vi "Read Line.vi"(8 "error in (no error)":errorcluster, 11 "Table Manager in":refnum<class "Table Manager.lvclass">) -> (0 "error out":errorcluster, 2 "Table Manager.lvlib:Line.lvclass":refnum<class "Line.lvclass">, 3 "Table Manager out":refnum<class "Table Manager.lvclass">)   [LabVIEW 2013, in "Table Manager.lvlib" / "Table Manager.lvclass"]
uses:
  Table Manager.lvclass
  Line/Line.lvclass
  Table Manager.lvclass/Table Manager.ctl
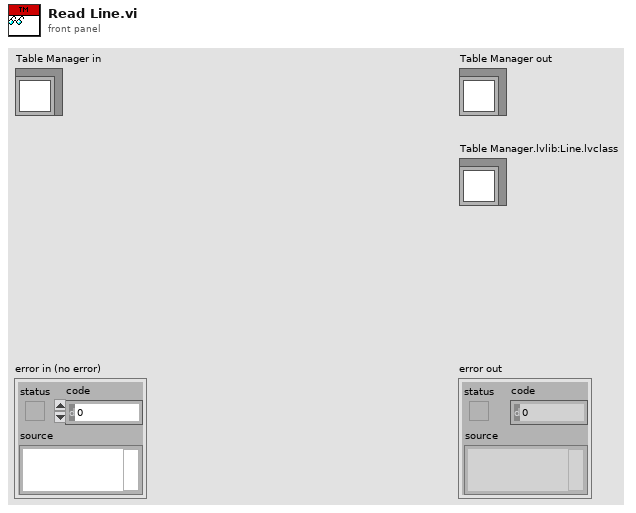
[diagram p1: front panel]
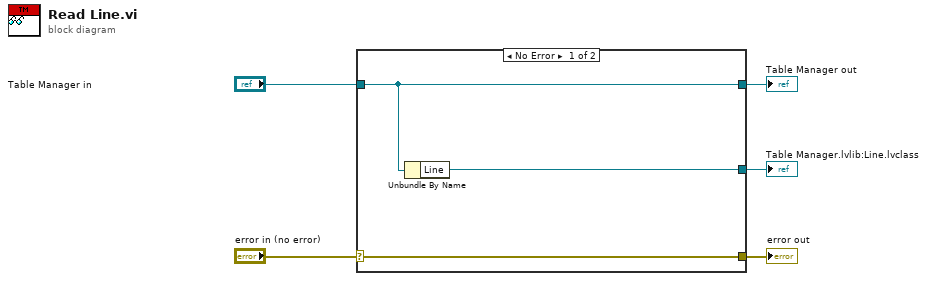
[diagram p0: block diagram]
diagram:
  n1 = case shown="No Error" "error in (no error)" {
    selector: "error in (no error)" -> [w8 w9]
    tunnel: [w8 w9] -> w4
    tunnel: [w7 w10] -> w2
    tunnel: "Table Manager in" -> [w7 w10]
    tunnel: [w6 _] -> w1
    frame No Error {
      n2 = Unbundle By Name(w7) -> ("Line"=w6:refnum<class "Line.lvclass">)
    }
    frame Error {
    }
  }
  "error out" <- w4
  "Table Manager out" <- w2
  "Table Manager.lvlib:Line.lvclass" <- w1
